vi "Generate LabVIEW FPGA Code for Multirate Filter.vi"() -> ()   [LabVIEW 2023]
doc: "Demonstrates how to use the DFD FXP MRate Code Generator VI to generate LabVIEW field-programmable gate array (FPGA) code from a fixed-point multirate filter.\n\nComplete the following steps to use this VI.\n1) Specify the <B>Quantization Settings</B> and <B>Modeling Settings</B>.\n2) Specify a <B>Destination Folder</B> for code generation.\n3) Specify a <B>Filter Name</B> for code generation.\n4) Specify <B># Channels</B> that you want the filter to process.\n5) Specify <B>Open Project?</B> to decide whether to open the generated LabVIEW project or not after code generation.\n6) Run the VI.\n7) Observe the Maximum Input Fs@40 MHz FPGA Clock to obtain information about the processing power of the generated fixed-point multirate filter block."
uses:
  <vilib>/addons/Digital Filter Design/Design.llb/DFD MRate Filter Design (Integer).vi
  <vilib>/addons/Digital Filter Design/NI_DigFilterLicensed.lvlib
panel:
  out "Maximum Input Fs@40 MHz FPGA Clock":dbl format="%#_5p Hz"
  out "lvproj Path":path
  in  "Open Project?":bool=TRUE
  in  "Filter Name":string
  in  "# Channels":i32=1
  in  "Destination Folder":path
  out "Error Message":string
  in  "Output Word Length":i16=16
  in  "Input Word Length":i16=16
  in  "Coefficients Word Length":i16=16
  # "Select Help>>Show Context Help and move the cursor over the VI icon for more information."
  # "Quantization Setting"
  # "Code Generation Settings"
  # "Code Generation Feedback"
  # "Modeling Settings"
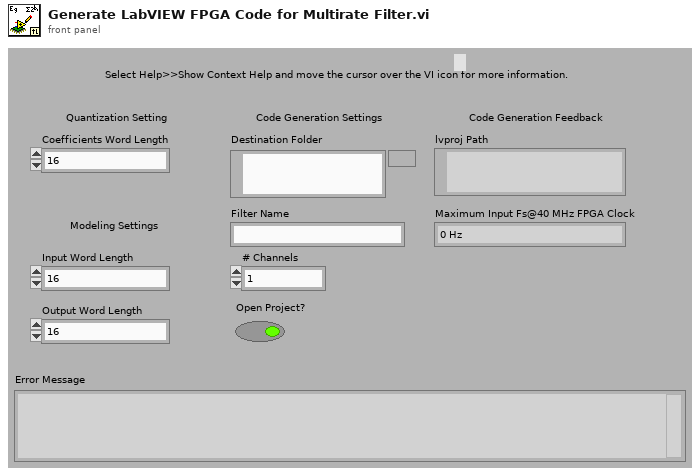
[diagram p1: front panel]
types:
  T1 = typedef "NI_DigFilterLicensed.lvlib/DFD Multirate Filter Obj.ctl" = cluster{"mMRate_Structure":enum16{"CIC", "FIR", "IIR", "Lattice"}, "mMRate_Mode":T2, "mMRate_Factor":i32, "mMRate_FIRParams":cluster{"mMRate_FIR_H":dbl[], "mMRate_FIR_IsNyquist?":bool, "mMRate_FIR_IsSymmetric?":bool}, "mMRate_CICParams":cluster{"mMRate_CIC_#Stage":i32, "mMRate_CIC_Lag":i32, "mMRate_CIC_Type":enum16{"Lowpass", "Highpass"}}, "mMRate_Order":i32, "mMRate_Version":string, "mMRate_Comments":string, "mMRate_RationalFactor":cluster{"mMRate_L":i32, "mMRate_M":i32}, "mMRate_Fs":dbl, "mMRate_Quantized?":bool, "mMRate_QFilterGain":dbl, "mMRate_CoefWl":i16, "mMRate_Scaling":cluster{"mMRate_ScaleByPowerOf2?":bool, "mMRate_ScaleType":T3}, "mMRate_InputWl":i16, "mMRate_OutputWl":i16, "mMRate_OutputMode":T4, "mMRate_MultMode":T5, "mMRate_BitPruning":bool, "mMRate_GainWl":i16, "mMRate_OutputFwl":i16, "mMRate_SumIwl":i16, "mMRate_InputIwl ":i16, "mMRate_SumWl":i16, "mMRate_CoefIwl":i16}
  T2 = typedef "NI_DigFilterLicensed.lvlib/DFD Multirate Mode.ctl" = i16
  T3 = typedef "NI_DigFilterLicensed.lvlib/DFD Coef Norm Type.ctl" = enum16{"No Norm", "Time Domain 1-Norm", "Time Domain 2-Norm", "Time Domain Inf-Norm"}
  T4 = typedef "NI_DigFilterLicensed.lvlib/DFD Round-off Mode.ctl" = enum16{"Nearest", "Truncation"}
  T5 = typedef "NI_DigFilterLicensed.lvlib/DFD FXP MRate Multiply Mode.ctl" = enum16{"Truncated", "Full"}
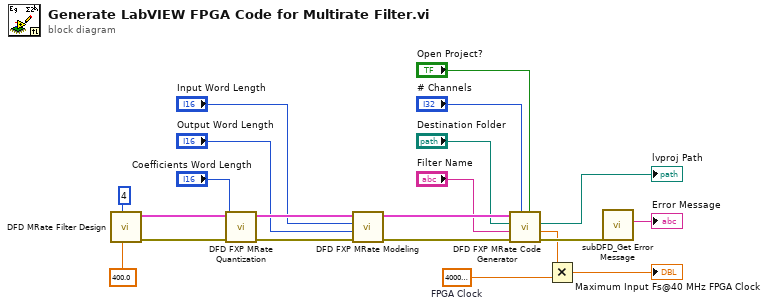
[diagram p0: block diagram]
diagram:
  w2 = 40000000.0  # FPGA Clock
  n1 = call-poly <vilib>:"DFD MRate Filter Design.vi"("fs in [Hz]"=400.0, "factor"=4) -> ("error out"=w20:errorcluster, "multirate filter out"=w21:T1)  [unwired: 6 in, 2 out]
  n2 = call <vilib>:"DFD FXP MRate Quantization.vi"("error in (no error)"=w20, "coefficients word length"="Coefficients Word Length", "multirate filter in"=w21) -> ("error out"=w15:errorcluster, "multirate filter out"=w17:T1)  [unwired: 3 in, 4 out]
  n3 = call <vilib>:"DFD FXP MRate Modeling.vi"("error in (no error)"=w15, "output word length"="Output Word Length", "input word length"="Input Word Length", "multirate filter in"=w17) -> ("error out"=w10:errorcluster, "multirate filter out"=w11:T1)  [unwired: 4 in, 2 out]
  n4 = call <vilib>:"DFD FXP MRate Code Generator.vi"("open project? (F)"="Open Project?", "# channels"="# Channels", "error in (no error)"=w10, "filter name"="Filter Name", "destination folder"="Destination Folder", "multirate filter"=w11) -> ("error out"=w9:errorcluster, "sampling frequency/FPGA clock"=w3:dbl, "lvproj path"=→"lvproj Path":path)  [unwired: 1 in, 2 out]
  n5 = Multiply(x=w3, y=w2) -> (x*y=→"Maximum Input Fs@40 MHz FPGA Clock":dbl)
  n6 = call <vilib>:"subDFD_Get Error Message.vi"("error in (no error)"=w9) -> ("Error Message"=→"Error Message":string)  [unwired: 10 out]
